vi "New.vi"(8 "error in (no error)":errorcluster, 11 "reference in":refnum<class "JTAG_Base.lvclass">) -> (0 "error out":errorcluster, 3 "reference out":refnum<class "JTAG_Base.lvclass">)   [LabVIEW 2022 SP3, in "JTAG_Base.lvlib" / "JTAG_Base.lvclass"]
uses:
  JTAG_Base.lvclass
  ObjectAttributes.ctl
  Config.ctl
  JTAG_Base.lvclass/JTAG_Base.ctl
  Components/ViPER.lvlibp/ViPER.lvclass
panel:
  in  "Data":T1
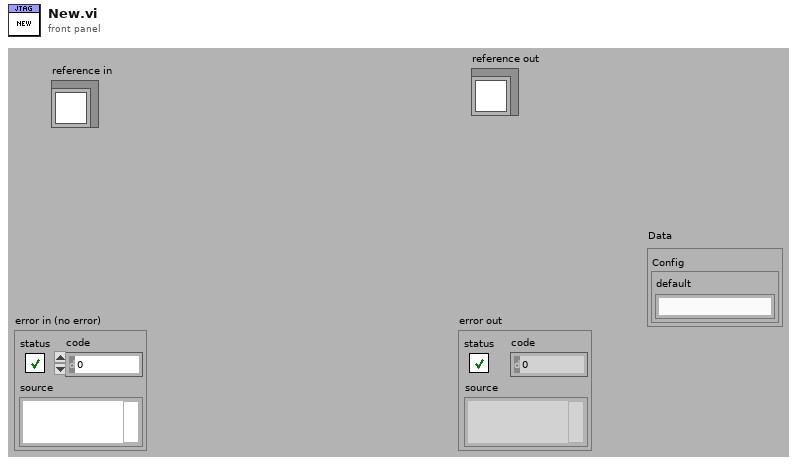
[diagram p1: front panel]
types:
  T1 = typedef "JTAG_Base.lvlib/JTAG_Base.lvclass/ObjectAttributes.ctl" = cluster{"Config":T2}
  T2 = typedef "JTAG_Base.lvlib/JTAG_Base.lvclass/Config.ctl" = cluster{"default":string}
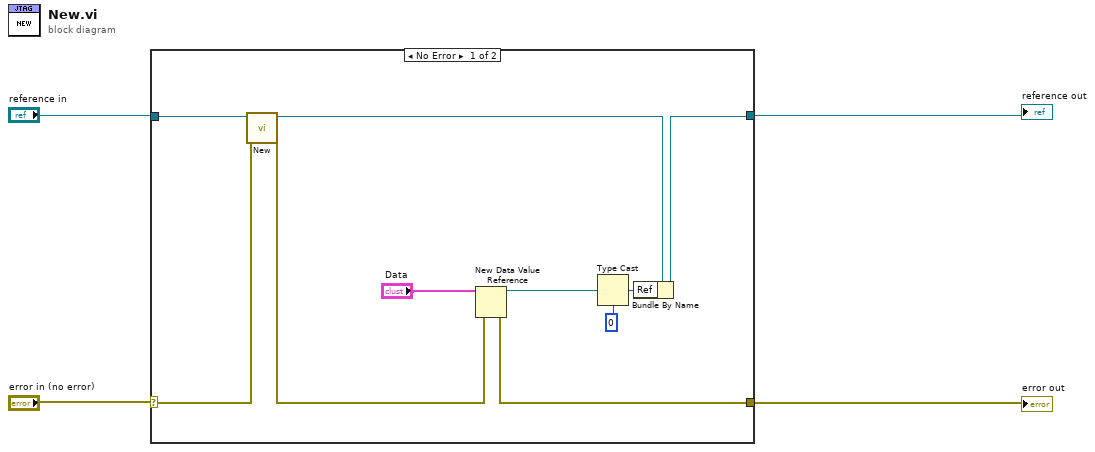
[diagram p0: block diagram]
diagram:
  n1 = case shown="No Error" "error in (no error)" {
    selector: "error in (no error)" -> [w14 w16]
    tunnel: [w13 w16] -> w2
    tunnel: "reference in" -> [w12 w15]
    tunnel: [w11 w15] -> w1
    frame No Error {
      n2 = call-parent "New.vi"("error in (no error)"=w14, "reference in"=w12) -> ("error out"=w5:errorcluster, "reference out"=w10:refnum<class "JTAG_Base.lvclass">)  [unwired: 8 in]
      n3 = New Data Value Reference(data value="Data", error in=w5) -> (data value reference=w8:refnum<data-value>, error out=w13:errorcluster)
      n4 = Type Cast(type=u32 0 ("DataRef"), x=w8) -> (*(type *) &x=w7:u32)
      n5 = Bundle By Name(cluster=w10, "Ref"=w7) -> (w11:refnum<class "JTAG_Base.lvclass">)
    }
    frame Error {
    }
  }
  "error out" <- w2
  "reference out" <- w1
